vi "SENS_FOM_RANG_SWE_TYPE.vi"(0 "VISA IN":refnum<visa-resource-name>, 1 "Range number":i32, 2 "Sweep Type":string(combo), 5 "error in":errorcluster, 7 "Channel":i32) -> (14 "VISA Out":refnum<visa-resource-name>, 19 "error out":errorcluster)   [LabVIEW 2018, in "PNA-X.lvlib"]
doc: "SENSe<cnum>:FOM:RANGe<n>:SWEep:TYPE <char> \n(Read-Write) Sets and returns the sweep type to be used with the specified range. \nThis setting is valid only if the specified range is already uncoupled from the primary range. \nLearn about Unsupported Sweep Type combinations. \nParameters \n<cnum> Any existing channel number; if unspecified, value is set to 1. \n<n> Range number. If unspecified, value is set to 1. \n<char> Sweep type. Choose from: \nCW - Also specify CW frequency. \nLINear - Also specify frequency Start/Stop or Center/Span \nLOG - Also specify frequency Start/Stop or Center/Span \nPOWer - Also specify power Start/Stop or Center/Span \nSEGMent - Also specify segment sweep settings. \n1742\n\nExamples SENS:FOM:RANG:SWE:TYPE LOG \nsense2:fom:range2:sweep:type linear: \nQuery Syntax SENSe<cnum>:FOM:RANGe<n>:SWEep:TYPE? \nReturn Type Character \nDefault Linear \nLast Modified: \n8-Mar-2007 MQX New topic \n1743\n\nSense:Frequency Commands \nSets the frequency sweep functions of the analyzer. \nClick on a blue keyword to view the command details. \nSee Also \nExample using some of these commands. \nLearn about Frequency Sweep \nSynchronizing the PNA and Controller \nSCPI Command Tree \nNote: All of the commands in this block will accept MIN or MAX instead of a numeric parameter. \nAlso, kHZ, MHz, and GHz are accepted as suffixes/units. \nSee SCPI Syntax for more information."
uses:
  PNA-X.lvlib
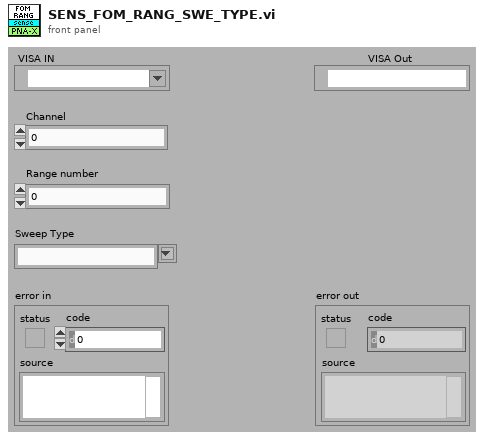
[diagram p1: front panel]
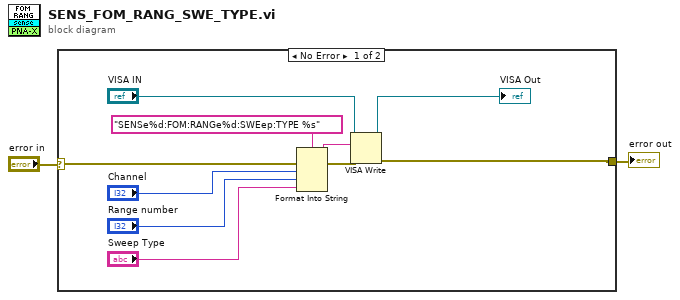
[diagram p0: block diagram]
diagram:
  n1 = case shown="No Error" "error in" {
    selector: "error in" -> [w12 w13]
    tunnel: [w7 w13] -> w1
    frame No Error {
      n2 = Format Into String(format string="SENSe%d:FOM:RANGe%d:SWEep:TYPE %s" ("Cmdline"), error in=w12, "Channel", "Range number", "Sweep Type") -> (resulting string=w10:string, error out=w11:errorcluster)  [unwired: 1 in]
      n3 = VISA Write(VISA resource name="VISA IN", write buffer=w10, error in (no error)=w11) -> (VISA resource name out=→"VISA Out":refnum<visa-resource-name>, error out=w7:errorcluster)  [unwired: 1 out]
    }
    frame Error {
    }
  }
  "error out" <- w1
